vi "Shutdown Sequence.vi"(7 "QRD":T1, 8 "error in":errorcluster, 11 "Loop ID":string) -> (0 "error out":errorcluster, 5 "QRD Out":T1)   [LabVIEW 2025]
uses:
  Controls/Queues-Refs-Data.ctl
  Builds/Queue Wrappers.lvlibp/Q Packet.ctl
  Builds/Queue Wrappers.lvlibp
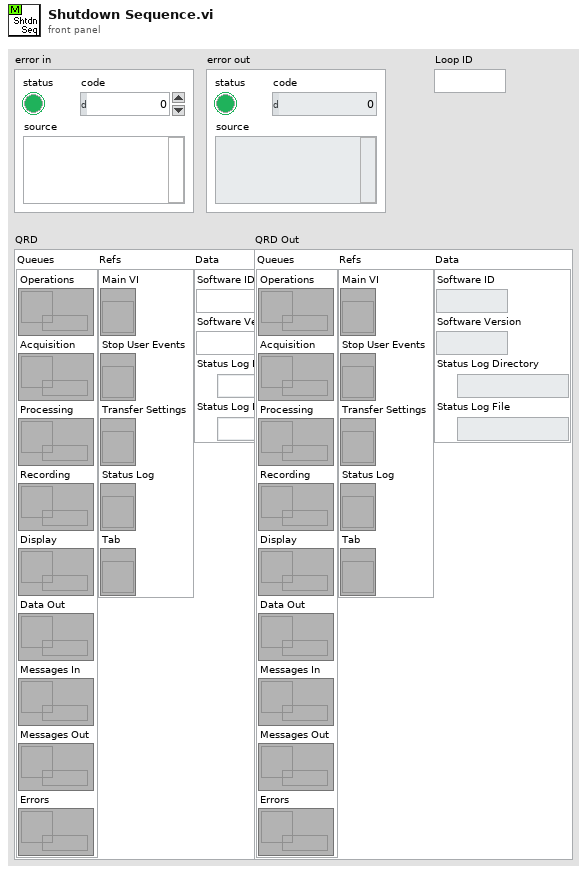
[diagram p1: front panel]
types:
  T1 = typedef "Queues-Refs-Data.ctl" = cluster{"Queues":cluster{"Operations":refnum<queue>, "Acquisition":refnum<queue>, "Processing":refnum<queue>, "Recording":refnum<queue>, "Display":refnum<queue>, "Data Out":refnum<queue>, "Messages In":refnum<queue>, "Messages Out":refnum<queue>, "Errors":refnum<queue>}, "Refs":cluster{"Main VI":refnum<vi>, "Stop User Events":refnum<vi>, "Transfer Settings":refnum<vi>, "Status Log":refnum<vi>, "Tab":refnum<vi>}, "Data":cluster{"Software ID":string, "Software Version":string, "Status Log Directory":path, "Status Log File":path}}
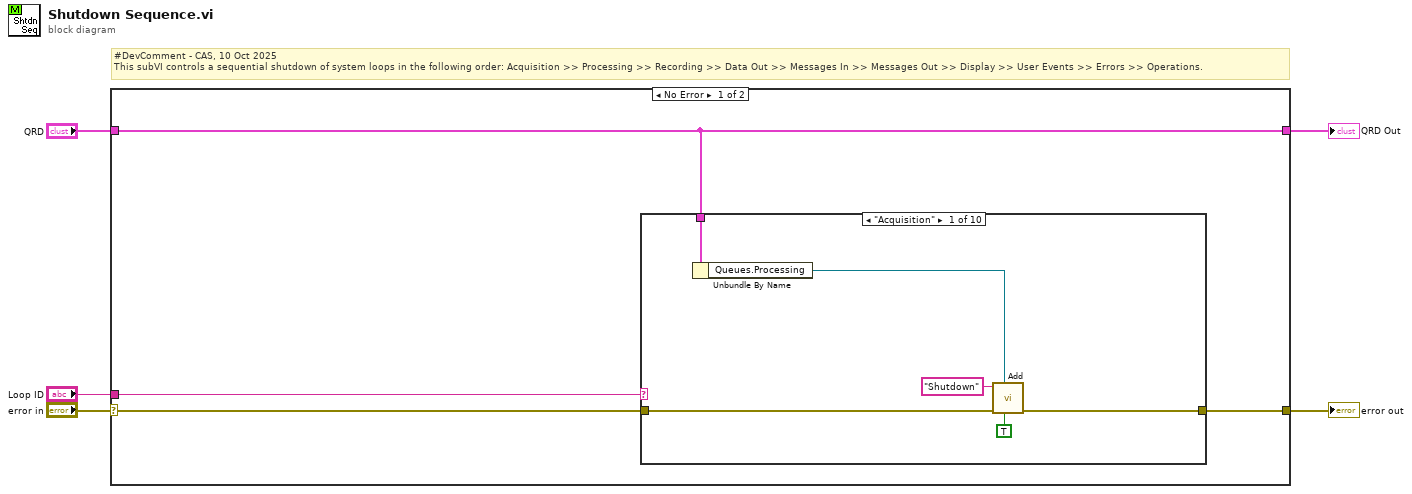
[diagram p0: block diagram]
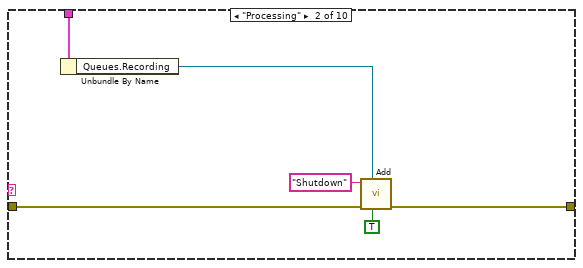
[diagram p2: hidden frame]
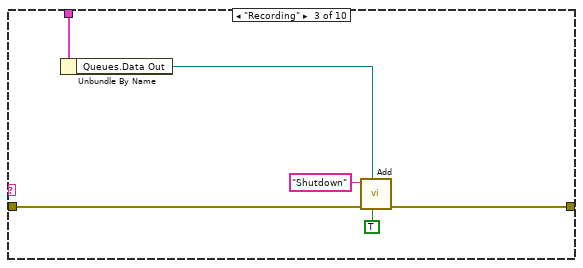
[diagram p3: hidden frame]
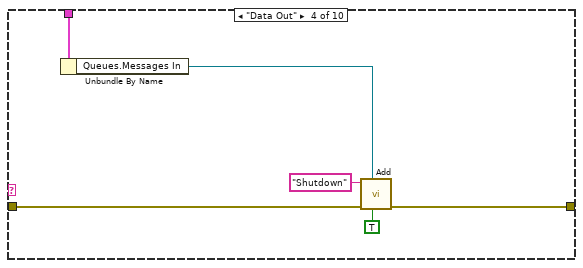
[diagram p4: hidden frame]
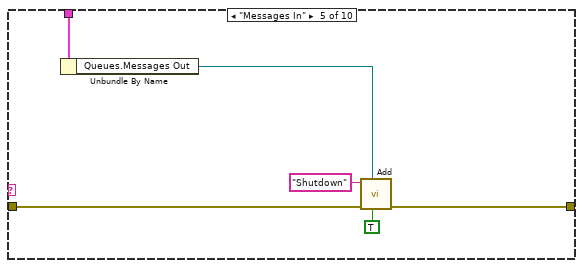
[diagram p5: hidden frame]
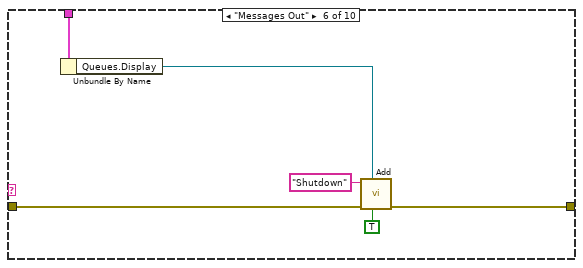
[diagram p6: hidden frame]
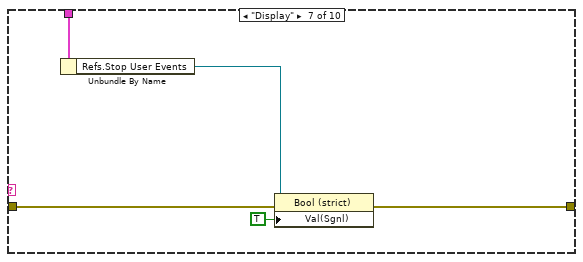
[diagram p7: hidden frame]
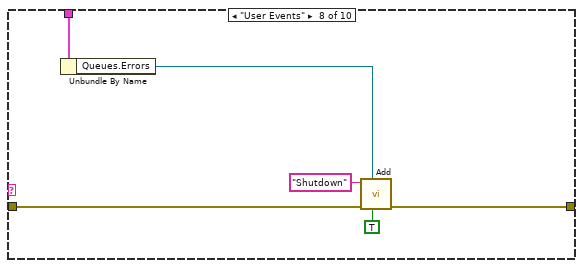
[diagram p8: hidden frame]
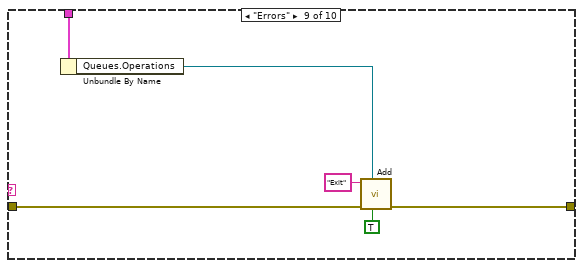
[diagram p9: hidden frame]
diagram:
  # "#DevComment - CAS, 10 Oct 2025\nThis subVI controls a sequential shutdown of system loops in the following order: Acquisition >> Processing >> Recording >> Data Out >> Messages In >> Messages Out >> Display >> User Events >> Errors >> Operations."
  n1 = case shown="No Error" "error in" {
    selector: "error in" -> [w7 w65]
    tunnel: [w6 w65] -> w4
    tunnel: [w9 w64] -> w3
    tunnel: "QRD" -> [w9 w64]
    tunnel: "Loop ID" -> [w8 _]
    frame No Error {
      n2 = case shown="\"Acquisition\"" w8 {
        tunnel: w9 -> [w15 w21 w27 w33 w39 w45 w50 w56 w62 _]
        tunnel: w7 -> [w14 w20 w26 w32 w38 w44 w47 w55 w61 w63]
        tunnel: [w13 w19 w25 w31 w37 w43 w46 w54 w60 w63] -> w6
        frame "Acquisition" {
          n3 = Unbundle By Name(w15) -> ("Queues.Processing"=w12:refnum<queue>)
          n4 = call "Add.vi"("Priority Message"=TRUE, "Q Ref In"=w12, "error in"=w14, "Packet ID"="Shutdown") -> ("error out"=w13:errorcluster)  [unwired: 4 in, 3 out]
        }
        frame "Processing" {
          n5 = Unbundle By Name(w21) -> ("Queues.Recording"=w18:refnum<queue>)
          n6 = call "Add.vi"("Priority Message"=TRUE, "Q Ref In"=w18, "error in"=w20, "Packet ID"="Shutdown") -> ("error out"=w19:errorcluster)  [unwired: 4 in, 3 out]
        }
        frame "Recording" {
          n7 = Unbundle By Name(w27) -> ("Queues.Data Out"=w24:refnum<queue>)
          n8 = call "Add.vi"("Priority Message"=TRUE, "Q Ref In"=w24, "error in"=w26, "Packet ID"="Shutdown") -> ("error out"=w25:errorcluster)  [unwired: 4 in, 3 out]
        }
        frame "Data Out" {
          n9 = Unbundle By Name(w33) -> ("Queues.Messages In"=w30:refnum<queue>)
          n10 = call "Add.vi"("Priority Message"=TRUE, "Q Ref In"=w30, "error in"=w32, "Packet ID"="Shutdown") -> ("error out"=w31:errorcluster)  [unwired: 4 in, 3 out]
        }
        frame "Messages In" {
          n11 = Unbundle By Name(w39) -> ("Queues.Messages Out"=w36:refnum<queue>)
          n12 = call "Add.vi"("Priority Message"=TRUE, "Q Ref In"=w36, "error in"=w38, "Packet ID"="Shutdown") -> ("error out"=w37:errorcluster)  [unwired: 4 in, 3 out]
        }
        frame "Messages Out" {
          n13 = Unbundle By Name(w45) -> ("Queues.Display"=w42:refnum<queue>)
          n14 = call "Add.vi"("Priority Message"=TRUE, "Q Ref In"=w42, "error in"=w44, "Packet ID"="Shutdown") -> ("error out"=w43:errorcluster)  [unwired: 4 in, 3 out]
        }
        frame "Display" {
          n15 = Unbundle By Name(w50) -> ("Refs.Stop User Events"=w49:refnum<vi>)
          n16 = property class="Bool (strict)"(reference=w49, error in=w47, "Val(Sgnl)"=TRUE ("Value (Signaling)")) -> (error out=w46:errorcluster)  [unwired: 1 out]
        }
        frame "User Events" {
          n17 = Unbundle By Name(w56) -> ("Queues.Errors"=w53:refnum<queue>)
          n18 = call "Add.vi"("Priority Message"=TRUE, "Q Ref In"=w53, "error in"=w55, "Packet ID"="Shutdown") -> ("error out"=w54:errorcluster)  [unwired: 4 in, 3 out]
        }
        frame "Errors" {
          n19 = Unbundle By Name(w62) -> ("Queues.Operations"=w59:refnum<queue>)
          n20 = call "Add.vi"("Priority Message"=TRUE, "Q Ref In"=w59, "error in"=w61, "Packet ID"="Exit") -> ("error out"=w60:errorcluster)  [unwired: 4 in, 3 out]
        }
        frame Default {
        }
      }
    }
    frame Error {
    }
  }
  "error out" <- w4
  "QRD Out" <- w3
